vi "subvi Robot Tile Count.vi"(3 "OverlapPriority":bool, 4 "TileLength":dbl, 5 "MinOverlap":dbl, 6 "MotorTravel":dbl) -> (0 "EdgelLength":dbl, 1 "ActualOverlap":dbl, 2 "NumTiles":u32)   [LabVIEW 2012]
panel:
  # "Inputs"
  # "Outputs"
  # "By default, number of tiles are calculated so that edge length is preserved.\nActual overlap may be greater than minimum.\nBut if overlap priority is desired, than overlap will be as specified but\nedge length covered by tiles will be greater."
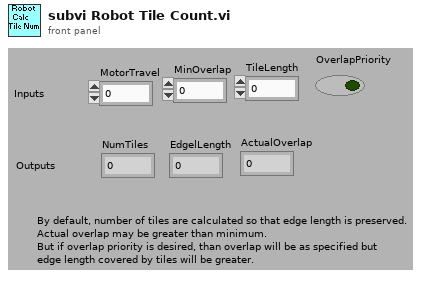
[diagram p1: front panel]
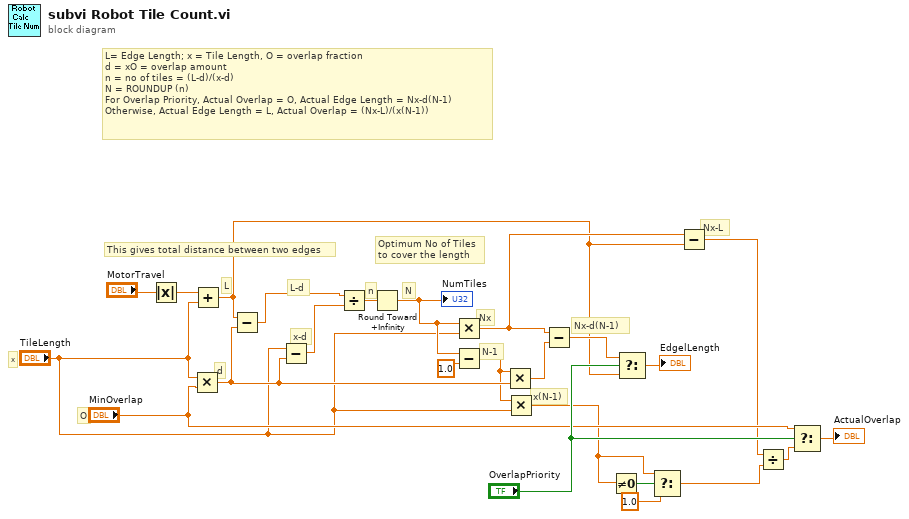
[diagram p0: block diagram]
diagram:
  # "x(N-1)"
  # "Nx-L"
  # "Nx-d(N-1)"
  # "N-1"
  # "Nx"
  # "N"
  # "n"
  # "x-d"
  # "L-d"
  # "d"
  # "O"
  # "x"
  # "L"
  # "L= Edge Length; x = Tile Length, O = overlap fraction\nd = xO = overlap amount\nn = no of tiles = (L-d)/(x-d)\nN = ROUNDUP (n)\nFor Overlap Priority, Actual Overlap = O, Actual Edge Length = Nx-d(N-1)\nOtherwise, Actual Edge Length = L, Actual Overlap = (Nx-L)/(x(N-1))"
  # "Optimum No of Tiles\nto cover the length"
  # "This gives total distance between two edges"
  n1 = Absolute Value(x="MotorTravel") -> (abs(x)=w22:dbl)
  n2 = Multiply(x="TileLength", y="MinOverlap") -> (x*y=w14:dbl)
  n3 = Add(x=w22, y="TileLength") -> (x+y=w9:dbl)
  n4 = Subtract(x=w9, y=w14) -> (x-y=w18:dbl)
  n5 = Subtract(x="TileLength", y=w14) -> (x-y=w17:dbl)
  n6 = Divide(x=w18, y=w17) -> (x/y=w24:dbl)
  n7 = Round Toward +Infinity(x=w24) -> (ceil(x): smallest int >= x=w16:dbl)
  "NumTiles" <- w16
  n8 = Multiply(x=w16, y="TileLength") -> (x*y=w10:dbl)
  n9 = Subtract(x=w16, y=1.0 ("x")) -> (x-y=w7:dbl)
  n10 = Multiply(x=w7, y=w14) -> (x*y=w13:dbl)
  n11 = Multiply(x=w7, y="TileLength") -> (x*y=w3:dbl)
  n12 = Subtract(x=w10, y=w13) -> (x-y=w12:dbl)
  n13 = Not Equal To 0?(x=w3) -> (x != 0?=w4:bool)
  n14 = Select(t=w12, s="OverlapPriority", f=w9) -> (s? t:f=→"EdgelLength":dbl)
  n15 = Select(t=w3, s=w4, f=1.0) -> (s? t:f=w1:dbl)
  n16 = Subtract(x=w10, y=w9) -> (x-y=w6:dbl)
  n17 = Divide(x=w6, y=w1) -> (x/y=w5:dbl)
  n18 = Select(t="MinOverlap", s="OverlapPriority", f=w5) -> (s? t:f=→"ActualOverlap":dbl)
